vi "Pre Launch Init.vi"(11 "Storage in":refnum<class "Storage.lvclass">) -> (0 "error out":errorcluster, 3 "Storage out":refnum<class "Storage.lvclass">)   [LabVIEW 2015, in "AMS UI.lvlib" / "Storage.lvclass"]
doc: "(<B>Filename</B>: Actor Framework.lvlib:Actor.lvclass:Pre Launch Init.vi)\n\nDefines behavior that occurs after the Launch Actor method is invoked but before the actor's Actor Core method begins running.\n\nThe Pre Launch Init method is guaranteed to finish before the Launch Actor method returns to its caller and before the actor itself receives any messages. Any references that the Pre Launch Init method obtains are guaranteed to have the same lifetime as the actor itself. Any errors that the Pre Launch Init method returns will abort the launch.\n\nBy default, this method does nothing. A descendant class may override it to define behavior."
uses:
  Storage.lvclass
  eActor Messages/Timeout Msg/Timeout Msg.lvclass
  <vilib>/ActorFramework/Message Enqueuer/Message Priority.ctl
  Controls/Register For Notifications Enumerator.ctl
  Storage.lvclass/Storage.ctl
  AMS Gas Actor/AMS Gas Actor.lvclass
  <vilib>/ActorFramework/Message Enqueuer/Message Enqueuer.lvclass
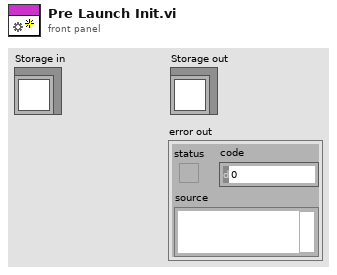
[diagram p1: front panel]
types:
  T1 = typedef "Register For Notifications Enumerator.ctl" = enum16{"Storage Tubes", "Storage Valves", "Sample Lines", "Syringe Container", "Capillary Container", "Preparation Line"}
  T2 = cluster{"Read Access":enum8{"Allowed", "Required", "None"}, "Write Access":enum8{"Allowed", "Required", "None"}}
  T3 = typedef "Actor Framework.lvlib/Message Enqueuer.lvclass/Message Priority.ctl" = enum16{"Low", "Normal", "High"}
  T4 = typedef "Sample Container.ctl" = cluster{"Sample In":refnum<k21>, "Sample Name":refnum<k21>, "Ti Cathode":refnum<k21>, "SampleQ":refnum<queue>}
  T5 = typedef "FP Control Refs Cluster.ctl" = cluster{"Liquid N Valve References":T6, "Main Line Valve Refs":T7, "Transfer Line Container":refnum<vi>, "Storage Containers":refnum<vi>[], "Sample Refs":T8, "Syringe Ctrl Refs ":T9, "Baratrons Chart":refnum<vi>, "Capillary Container":refnum<vi>, "Preparation Container":refnum<vi>, "Monkey Mode":refnum<vi>}
  T6 = typedef "Liquid N Valve Ref Cluster.ctl" = cluster{"Cold Bath H2O HV 100":refnum<vi>, "Cold Bath Cleaning HV 101":refnum<vi>, "Cold Bath Storage 1 HV 102":refnum<vi>, "Cold Bath Storage 2 HV 103":refnum<vi>, "Cold Bath Storage 3 HV 104":refnum<vi>, "Cold Bath Storage 4 HV 105":refnum<vi>, "Cold Bath Syringe HV 106":refnum<vi>, "Liquid N Master Valve HV 107":refnum<vi>}
  T7 = typedef "Main Line Valve Ref Cluster.ctl" = cluster{"Turbo Valve DV313":refnum<vi>, "Prep Line Valve 0 DV300":refnum<vi>, "Storage Valves":refnum<vi>[]}
  T8 = typedef "Sample Valve Refs.ctl" = cluster{"Valves":cluster{"Sample 5 DV318":refnum<vi>, "Sample 4 DV317":refnum<vi>, "Sample 3 DV316":refnum<vi>, "Sample 2 DV315":refnum<vi>, "Sample 1 DV314":refnum<vi>}, "Lines":cluster{"Sample 1":refnum<vi>, "Sample 2":refnum<vi>, "Sample 3":refnum<vi>, "Sample 4":refnum<vi>, "Sample 5":refnum<vi>}}
  T9 = typedef "Syringe Ctrl Refs.ctl" = cluster{"Syringe Home":refnum<vi>, "Syringe Freeze":refnum<vi>, "Syringe TC":refnum<vi>, "Syringe Container":refnum<vi>}
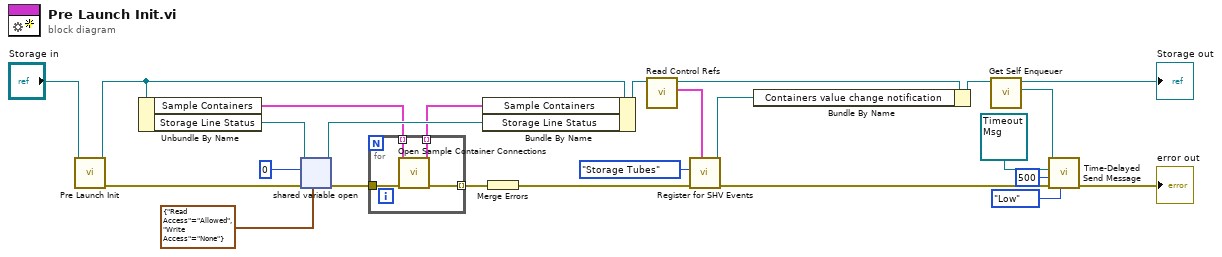
[diagram p0: block diagram]
diagram:
  n1 = call-parent "Pre Launch Init.vi"("eActor in"="Storage in") -> ("error out"=w17:errorcluster, "eActor out"=w18:refnum<class "Storage.lvclass">)  [unwired: 9 in]
  n2 = Unbundle By Name(w18) -> ("Sample Containers"=w10:T4[], "Storage Line Status"=w15:refnum<k21>)
  n3 = shared-variable-open(w15, w17, u16 0, T2 {"Read Access"=enum."Allowed", "Write Access"=enum."None"} ("access")) -> (w13:refnum<k21>, w12:errorcluster)
  n4 = for {
    tunnel: w12 -> [w29]
    tunnel: [w28] -> w11 mode=indexing
    tunnel: w10 -> [w27] mode=indexing
    tunnel: [w26] -> w9 mode=indexing
    n5 = call "Open Sample Container Connections.vi"("error in (no error)"=w29, "Container in"=w27) -> ("error out"=w28:errorcluster, "Container out"=w26:T4)  [unwired: 8 in]
  }
  n6 = Bundle By Name(cluster=w18, "Sample Containers"=w9, "Storage Line Status"=w13) -> (w6:refnum<class "Storage.lvclass">)
  n7 = Merge Errors(w11) -> (w8:errorcluster)
  n8 = call-dynamic "Read Control Refs.vi"("AMS Gas Actor in"=w6) -> ("Control Refs"=w4:T5, "AMS Gas Actor out"=w5:refnum<class "Storage.lvclass">)  [unwired: 9 in]
  n9 = call "Register for SHV Events.vi"("Control Refs"=w4, "error in (no error)"=w8, "Register for"=Register_For_Notifications_Enumerator."Storage Tubes") -> ("error out"=w7:errorcluster, "Containers SHV change notification"=w3:refnum<user-event>)  [unwired: 7 in]
  n10 = Bundle By Name(cluster=w5, "Containers value change notification"=w3) -> (w2:refnum<class "Storage.lvclass">)
  n11 = call-dynamic "Get Self Enqueuer.vi"("eActor in"=w2) -> ("Actor Framework:Message Enqueuer"=w22:refnum<class "Message Enqueuer.lvclass">, "eActor out"=→"Storage out":refnum<class "Storage.lvclass">)  [unwired: 9 in]
  n12 = call <vilib>:"Time-Delayed Send Message.vi"("Message Priority (Normal)"=Message_Priority."Low", "error in (no error)"=w7, "Milliseconds To Wait"=500, "Message"=refnum<class "Timeout Msg.lvclass"> refnum ("Timeout Msg.lvclass"), "Message Enqueuer"=w22) -> ("error out"=→"error out":errorcluster)  [unwired: 5 in, 1 out]
